vi "INITIALISATION.vi"(2 "error in (no error)":errorcluster, 5 "VISAcurrent source":refnum<visa-resource-name>="K2401") -> (3 "error out":errorcluster)   [LabVIEW 2019]
uses:
  <instrlib>/Keithley 24XX/Keithley 24XX.lvlib
  <instrlib>/Keithley 2182/Keithley 2182.lvlib
panel:
  out "VISA  nanoVM out":refnum<visa-resource-name>
  in  "VISAcnanovoltmeter":refnum<visa-resource-name>="nanovoltmeter"
  out "VISA current source out":refnum<visa-resource-name>
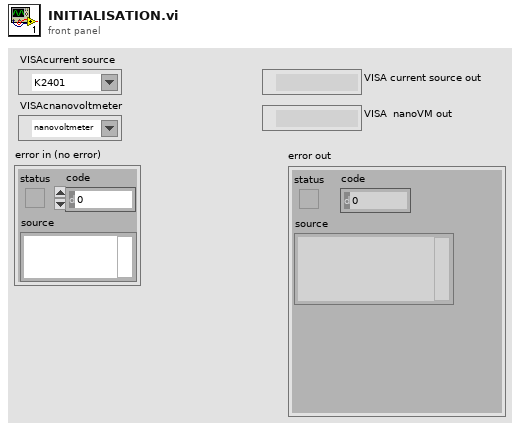
[diagram p1: front panel]
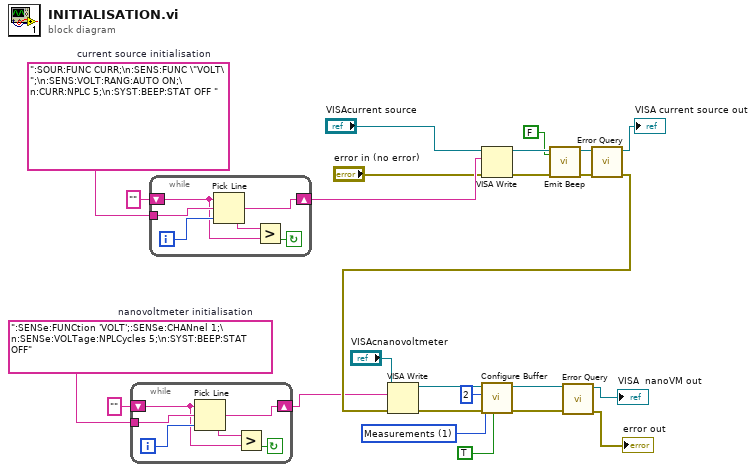
[diagram p0: block diagram]
diagram:
  w2 = 1 items=["None", "Measurements", "Math Calculation"] ("Buffer Source (0: None)")
  w13 = ":SENSe:FUNCtion 'VOLT';:SENSe:CHANnel 1;\n:SENSe:VOLTage:NPLCycles 5;\n:SYST:BEEP:STAT OFF"  # nanovoltmeter initialisation
  w24 = ":SOUR:FUNC CURR;\n:SENS:FUNC \"VOLT\";\n:SENS:VOLT:RANG:AUTO ON;\n:CURR:NPLC 5;\n:SYST:BEEP:STAT OFF "  # current source initialisation
  n1 = while {
    tunnel: w13 -> [w30]
    shift-right: [w26] -> w11
    shift-left: "" ("output string") -> [w27]
    i -> [w29]
    stop <- w28 continue-if-true
    n2 = Pick Line(string ("")=w27, multi-line string=w30, line index=w29) -> (output string=w26:string)
    n3 = Greater?(x=w26, y=w27) -> (0:w28:bool)
  }
  n4 = while {
    tunnel: w24 -> [w35]
    shift-right: [w31] -> w22
    shift-left: "" ("output string") -> [w32]
    i -> [w34]
    stop <- w33 continue-if-true
    n5 = Pick Line(string ("")=w32, multi-line string=w35, line index=w34) -> (output string=w31:string)
    n6 = Greater?(x=w31, y=w32) -> (0:w33:bool)
  }
  n7 = VISA Write(VISA resource name="VISAcurrent source", write buffer=w22, error in (no error)="error in (no error)") -> (VISA resource name out=w20:refnum<visa-resource-name>, error out=w19:errorcluster)  [unwired: 1 out]
  n8 = call <instrlib>:"Emit Beep.vi"("Enable Beep (F)"=FALSE, "error in (no error)"=w19, "VISA resource name"=w20) -> ("error out"=w18:errorcluster, "VISA resource name out"=w21:refnum<visa-resource-name>)  [unwired: 7 in]
  n9 = call <instrlib>:"Error Query.vi"("error in (no error)"=w18, "VISA resource name"=w21) -> ("error out"=w12:errorcluster, "VISA resource name out"=→"VISA current source out":refnum<visa-resource-name>)  [unwired: 6 in, 2 out]
  n10 = VISA Write(VISA resource name="VISAcnanovoltmeter", write buffer=w11, error in (no error)=w12) -> (VISA resource name out=w7:refnum<visa-resource-name>, error out=w5:errorcluster)  [unwired: 1 out]
  n11 = call <instrlib>:"Configure Buffer.vi"("Enable Buffer Statistics (0: Disable)"=TRUE, "error in (no error)"=w5, "Buffer Source (0: None)"=w2, "Buffer Size (2)"=2, "VISA resource name"=w7) -> ("error out"=w4:errorcluster, "VISA resource name out"=w6:refnum<visa-resource-name>)  [unwired: 5 in]
  n12 = call <instrlib>:"Error Query.vi"("error in (no error)"=w4, "VISA resource name"=w6) -> ("error out"=→"error out":errorcluster, "VISA resource name out"=→"VISA  nanoVM out":refnum<visa-resource-name>)  [unwired: 6 in, 2 out]
